vi "TimeStampNeeded.vi"(8 "Error In":errorcluster, 10 "Wvfrm_ref":T1={"t0"=timestamp(0 s since 1904-01-01), "dt"=1.0, "attributes"=variant, "Y_ref"=refnum} {"dt" format="%0.6f"; "t0" format="%<%X\n%x>T"}, 11 "Fitter In":refnum<class "FitterBase.lvclass">) -> (0 "Error Out":errorcluster, 1 "TsnGreaterThanSampleStart":bool, 2 "TsnLessThanSample Start Time":bool, 3 "Fitter Out":refnum<class "FitterBase.lvclass">, 4 "nSamplesNeeded":i32, 5 "TimeStampNeeded":ext)   [LabVIEW 2018, in "AnalysisPlugins.lvlib" / "FitterBase.lvclass"]
uses:
  FitterBase.lvclass
  Typedefs/clAnalysisConfig.ctl
  Digitizer/DigitizerPlugins/DigitizerBaseClass/Typedefs/WfrmAttributes.ctl
  Digitizer/DigitizerPlugins/DigitizerBaseClass/DigitizerBase.lvclass
  Typedefs/Wvfrm_ref.ctl
panel:
  out "AnalysisTime":timestamp
  out "SampleEndTime":timestamp
  out "SampleStartTime":timestamp
  out "TimeStampNeeded":timestamp
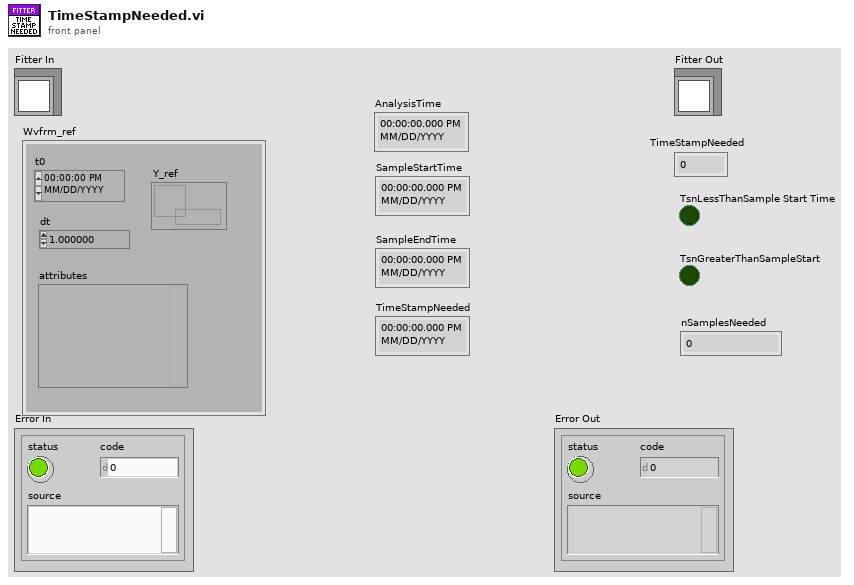
[diagram p1: front panel]
types:
  T1 = typedef "AnalysisPlugins.lvlib/FitterBase.lvclass/Wvfrm_ref.ctl" = cluster{"t0":timestamp, "dt":dbl, "attributes":variant, "Y_ref":refnum<data-value>}
  T2 = typedef "DigitizerPlugins.lvlib/DigitizerBase.lvclass/WfrmAttributes.ctl" = cluster{"XOffset":dbl, "ActualPts":i64, "FirstValid":i64}
  T3 = typedef "AnalysisPlugins.lvlib/FitterBase.lvclass/clAnalysisConfig.ctl" = cluster{"F0":u32, "SettlingTime":dbl, "AnalysisCycles":dbl, "SampleRate":dbl, "NumChannels":u32, "TsOffset":enum16{"start", "middle", "end"}}
  T4 = typedef "AnalysisPlugins.lvlib/AnalysisPluginsBase.lvclass/clWindowData.ctl" = cluster{"Timestamp":ext, "Samples":dbl[][], "Window Valid":bool, "T0":ext}
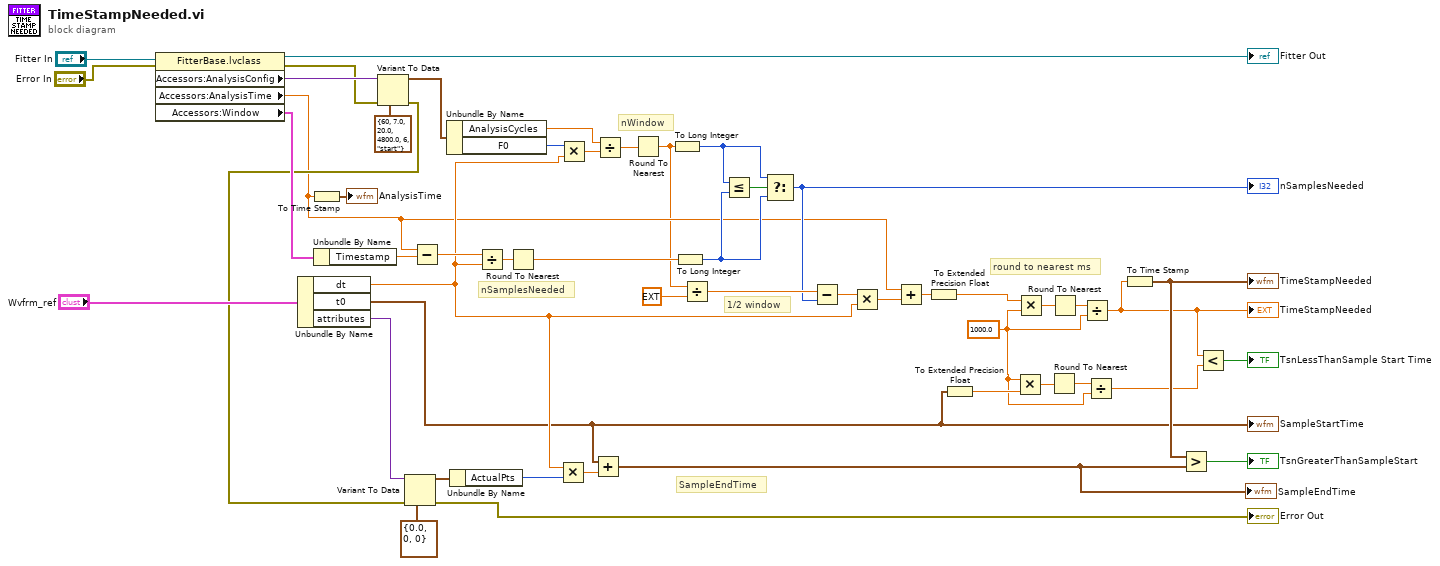
[diagram p0: block diagram]
diagram:
  w3 = 1000.0 ("y")
  # "1/2 window"
  # "SampleEndTime"
  # "round to nearest ms"
  # "nWindow"
  # "nSamplesNeeded"
  n1 = property class="FitterBase.lvclass"(reference="Fitter In", error in="Error In") -> (reference out=→"Fitter Out":refnum<class "FitterBase.lvclass">, error out=w48:errorcluster, "Accessors:AnalysisConfig"=w49:variant, "Accessors:AnalysisTime"=w10:dbl, "Accessors:Window"=w45:T4)
  n2 = Unbundle By Name("Wvfrm_ref") -> ("dt"=w21:dbl, "t0"=w7:timestamp, "attributes"=w26:variant)
  "SampleStartTime" <- w7
  n3 = To Time Stamp(1:w10) -> (0:→"AnalysisTime":timestamp)
  n4 = Unbundle By Name(w45) -> ("Timestamp"=w44:ext)
  n5 = Variant To Data(error in=w48, type=T3 {"F0"=60, "SettlingTime"=7.0, "AnalysisCycles"=20.0, "SampleRate"=4800.0, "NumChannels"=6, "TsOffset"=enum."start"} ("clAnalysisConfig"), Variant=w49) -> (data=w46:T3, error out=w25:errorcluster)
  n6 = Variant To Data(error in=w25, type=T2 {"XOffset"=0.0, "ActualPts"=0, "FirstValid"=0} ("Attributes"), Variant=w26) -> (data=w23:T2, error out=→"Error Out":errorcluster)
  n7 = Subtract(x=w10, y=w44) -> (x-y=w43:ext)
  n8 = Unbundle By Name(w46) -> ("AnalysisCycles"=w38:dbl, "F0"=w40:u32)
  n9 = Unbundle By Name(w23) -> ("ActualPts"=w22:i64)
  n10 = Divide(x=w43, y=w21) -> (x/y=w41:ext)
  n11 = Round To Nearest(number=w41) -> (nearest integer value=w35:ext)
  n12 = Multiply(x=w21, y=w22) -> (x*y=w20:dbl)
  n13 = Multiply(x=w40, y=w21) -> (x*y=w39:dbl)
  n14 = Add(x=w7, y=w20) -> (x+y=w17:timestamp)
  "SampleEndTime" <- w17
  n15 = Divide(x=w38, y=w39) -> (x/y=w37:dbl)
  n16 = Round To Nearest(number=w37) -> (nearest integer value=w8:dbl)
  n17 = To Long Integer(number=w8) -> (32bit integer=w12:i32)
  n18 = To Long Integer(number=w35) -> (32bit integer=w11:i32)
  n19 = Divide(x=w8, y=ext 2.0) -> (x/y=w33:ext)
  n20 = Less Or Equal?(x=w12, y=w11) -> (x <= y?=w36:bool)
  n21 = Select(t=w12, s=w36, f=w11) -> (s? t:f=w32:i32)
  "nSamplesNeeded" <- w32
  n22 = Subtract(x=w33, y=w32) -> (x-y=w31:ext)
  n23 = Multiply(x=w31, y=w21) -> (x*y=w30:ext)
  n24 = Add(x=w10, y=w30) -> (x+y=w29:ext)
  n25 = To Extended Precision Float(1:w29) -> (0:w13:ext)
  n26 = To Extended Precision Float(1:w7) -> (0:w6:ext)
  n27 = Multiply(x=w3, y=w6) -> (x*y=w5:ext)
  n28 = Multiply(x=w13, y=w3) -> (x*y=w28:ext)
  n29 = Round To Nearest(number=w5) -> (nearest integer value=w4:ext)
  n30 = Round To Nearest(number=w28) -> (nearest integer value=w27:ext)
  n31 = Divide(x=w27, y=w3) -> (x/y=w2:ext)
  "TimeStampNeeded" <- w2
  n32 = Divide(x=w4, y=w3) -> (x/y=w1:ext)
  n33 = To Time Stamp(1:w2) -> (0:w16:timestamp)
  "TimeStampNeeded" <- w16
  n34 = Greater?(x=w16, y=w17) -> (0:→"TsnGreaterThanSampleStart":bool)
  n35 = Less?(x=w2, y=w1) -> (x < y?=→"TsnLessThanSample Start Time":bool)
